vi "Get LV App Version And Name.vi"(11 "LabVIEW._Application":refnum<k7>) -> (0 "error out":errorcluster, 2 "AppName":string, 3 "Version":string)   [LabVIEW 2012]
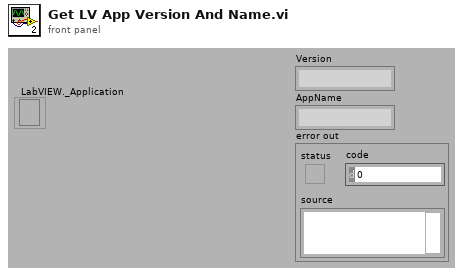
[diagram p1: front panel]
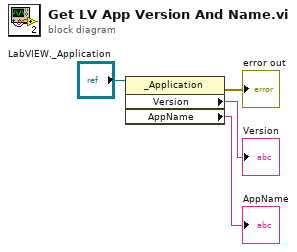
[diagram p0: block diagram]
diagram:
  n1 = property class="_Application"(reference="LabVIEW._Application") -> (error out=→"error out":errorcluster, "Version"=→"Version":string, "AppName"=→"AppName":string)  [unwired: 1 in, 1 out]
